vi "GetParticleResultValue.vi"(8 "error in (no error)":errorcluster, 9 "Data":T1, 11 "Analysis_Particle_Parameter":T2={"Selected Particle"=0, "Connectivity 4/8 (8)"=TRUE, "MaxParticle"=0}) -> (0 "error out":errorcluster, 3 "ResultValues":string[](array[string]))   [LabVIEW 2019]
uses:
  Controls/Particle/Analysis_Particle_Parameter.ctl
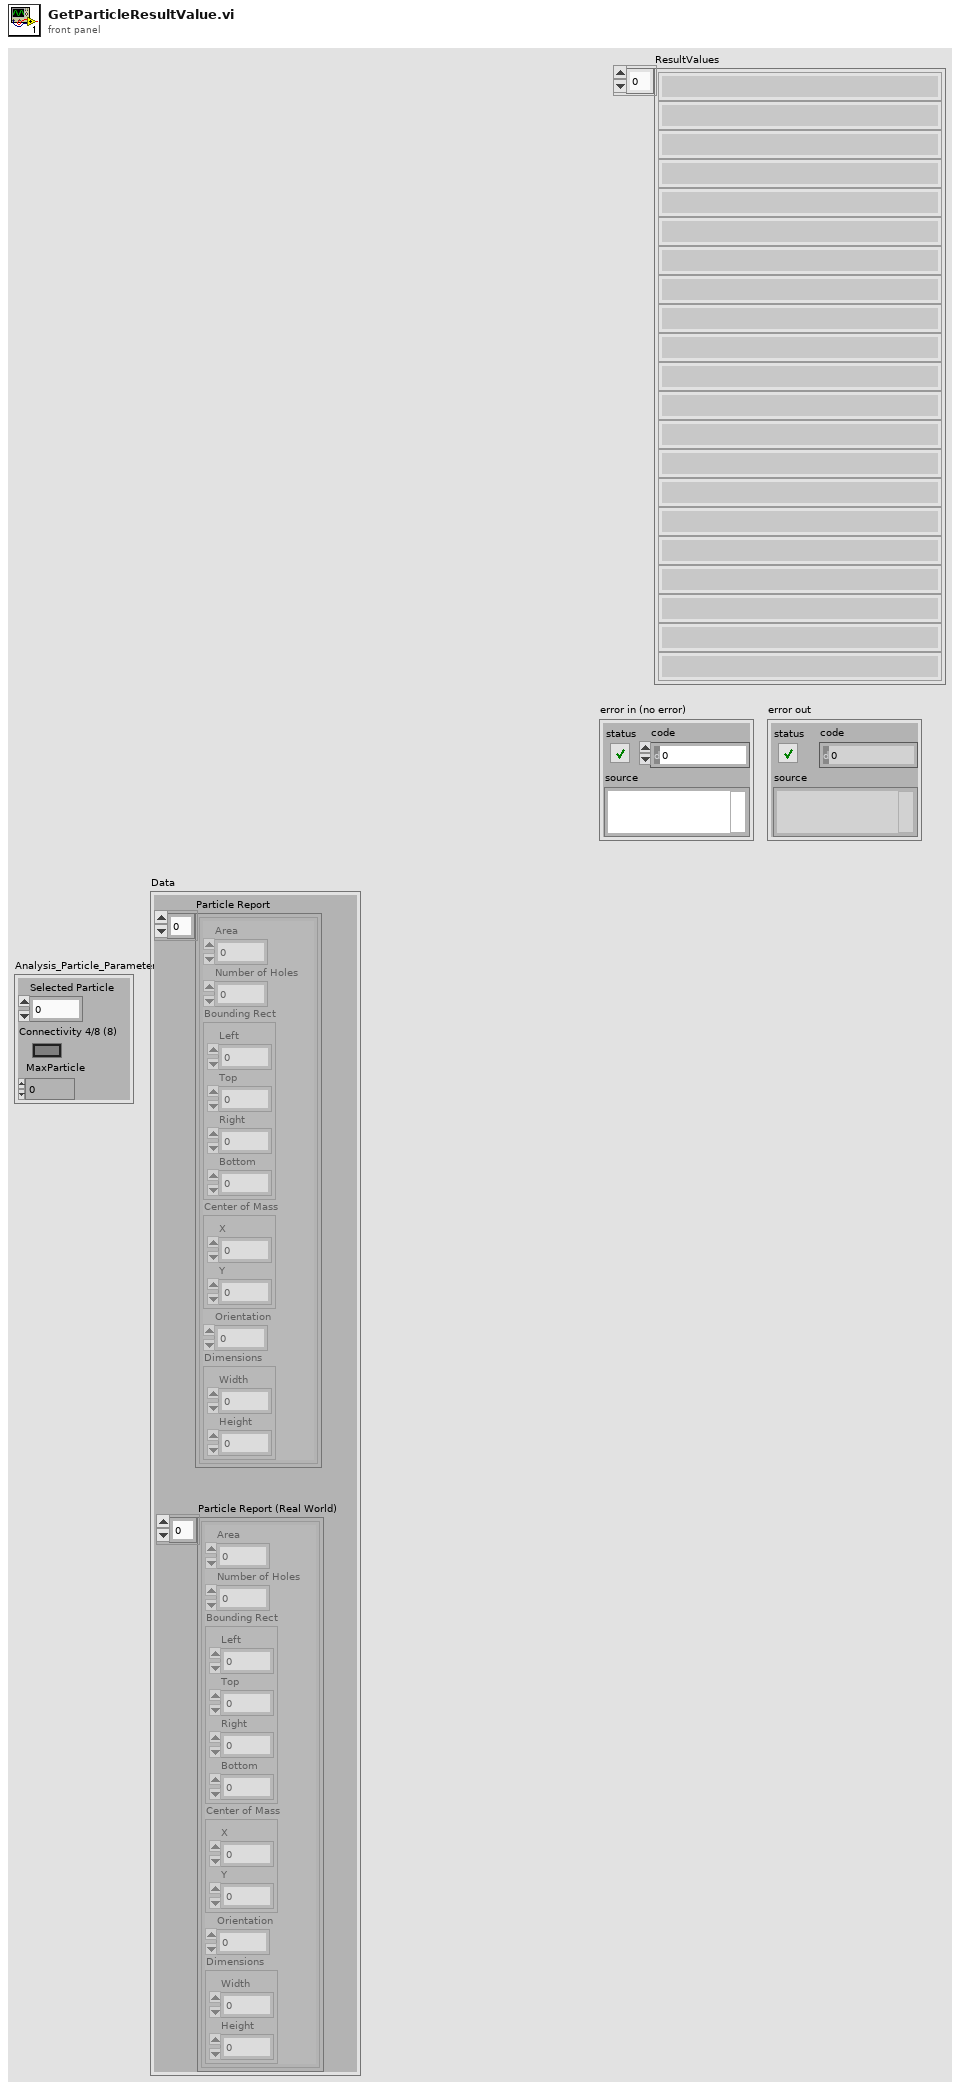
[diagram p1: front panel]
types:
  T1 = cluster{"Particle Report":cluster{"Area":dbl, "Number of Holes":dbl, "Bounding Rect":cluster{"Left":dbl, "Top":dbl, "Right":dbl, "Bottom":dbl}, "Center of Mass":cluster{"X":dbl, "Y":dbl}, "Orientation":dbl, "Dimensions":cluster{"Width":dbl, "Height":dbl}}[], "Particle Report (Real World)":cluster{"Area":dbl, "Number of Holes":dbl, "Bounding Rect":cluster{"Left":dbl, "Top":dbl, "Right":dbl, "Bottom":dbl}, "Center of Mass":cluster{"X":dbl, "Y":dbl}, "Orientation":dbl, "Dimensions":cluster{"Width":dbl, "Height":dbl}}[]}
  T2 = typedef "Analysis_Particle_Parameter.ctl" = cluster{"Selected Particle":i32, "Connectivity 4/8 (8)":bool, "MaxParticle":i32}
  T3 = cluster{"Area":dbl, "Number of Holes":dbl, "Bounding Rect":cluster{"Left":dbl, "Top":dbl, "Right":dbl, "Bottom":dbl}, "Center of Mass":cluster{"X":dbl, "Y":dbl}, "Orientation":dbl, "Dimensions":cluster{"Width":dbl, "Height":dbl}}[]
  T4 = cluster{"Left":dbl, "Top":dbl, "Right":dbl, "Bottom":dbl}
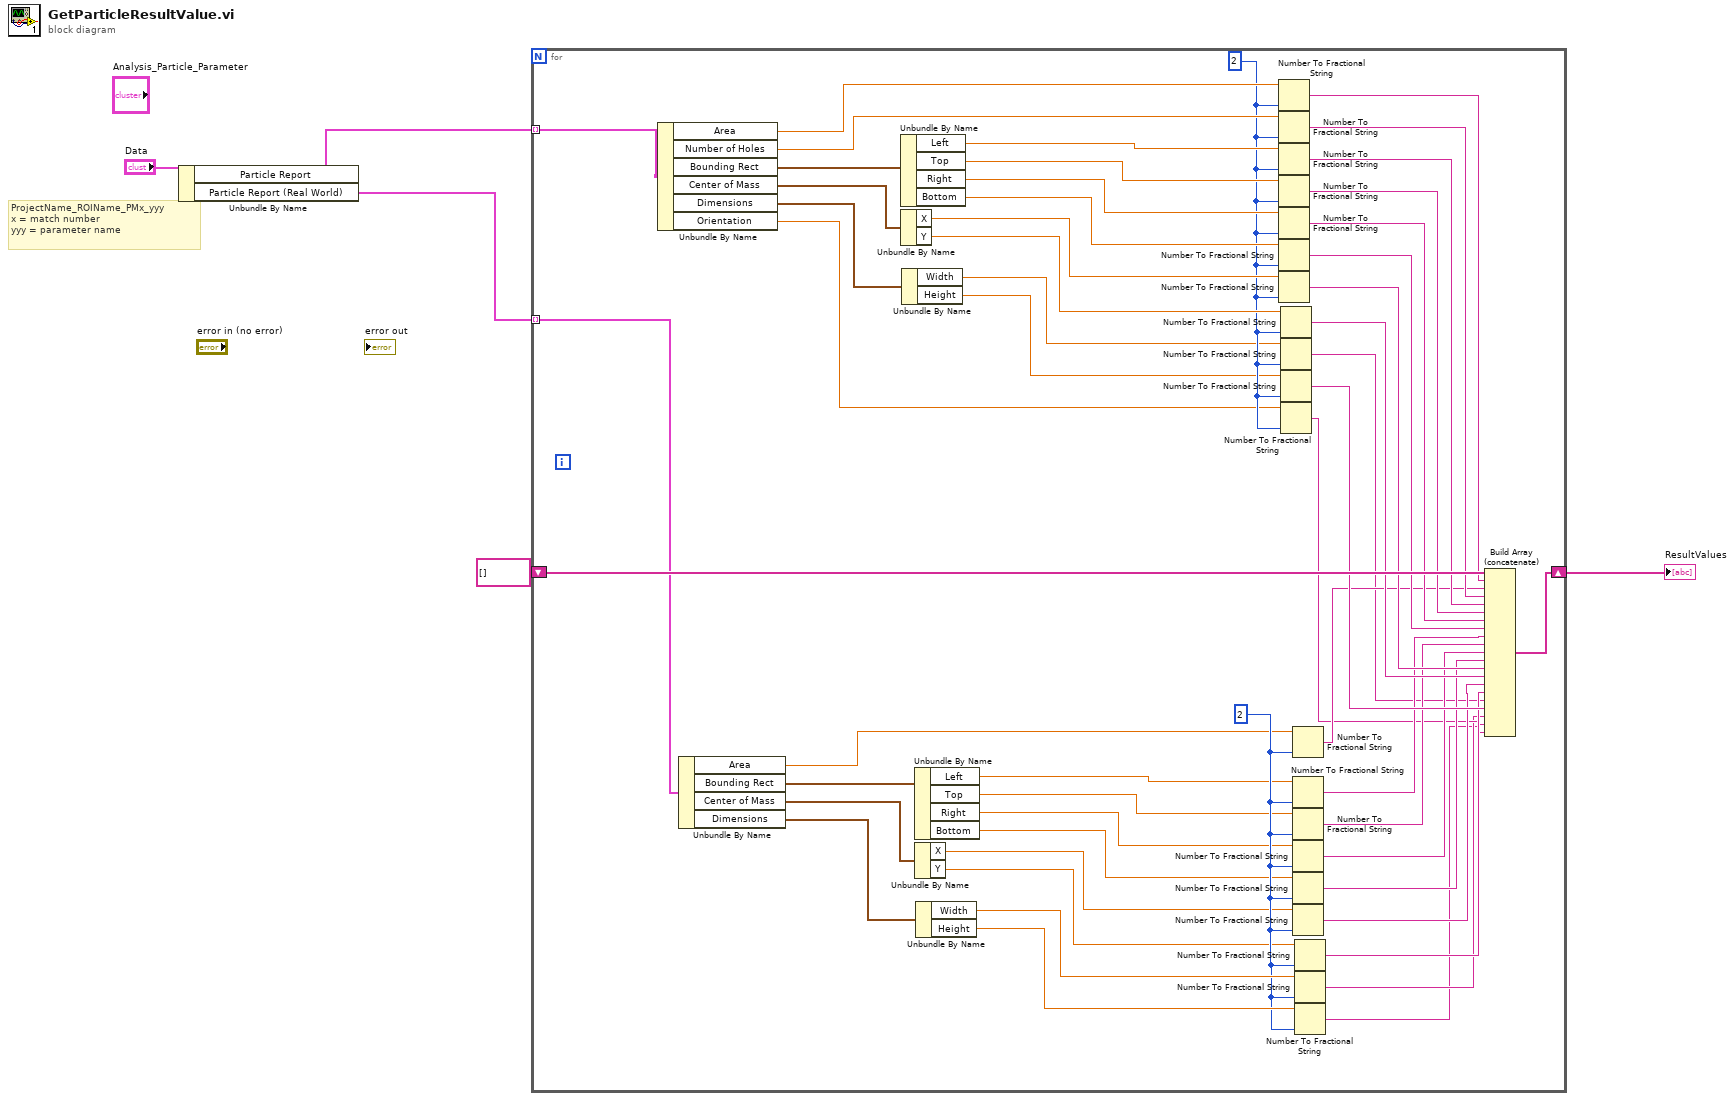
[diagram p0: block diagram]
diagram:
  # "ProjectName_ROIName_PMx_yyy\nx = match number\nyyy = parameter name"
  n1 = Unbundle By Name("Data") -> ("Particle Report"=w2:T3, "Particle Report (Real World)"=w1:T3)
  n2 = for {
    shift-right: [w31] -> w4
    shift-left: string[] [] -> [w57]
    tunnel: w2 -> [w41] mode=indexing
    tunnel: w1 -> [w17] mode=indexing
    w27 = 2
    w46 = 2
    n3 = Unbundle By Name(w41) -> ("Area"=w54:dbl, "Number of Holes"=w53:dbl, "Bounding Rect"=w56:T4, "Center of Mass"=w55:cluster{"X":dbl, "Y":dbl}, "Dimensions"=w45:cluster{"Width":dbl, "Height":dbl}, "Orientation"=w42:dbl)
    n4 = Unbundle By Name(w17) -> ("Area"=w20:dbl, "Bounding Rect"=w18:T4, "Center of Mass"=w19:cluster{"X":dbl, "Y":dbl}, "Dimensions"=w28:cluster{"Width":dbl, "Height":dbl})
    n5 = Unbundle By Name(w56) -> ("Left"=w52:dbl, "Top"=w51:dbl, "Right"=w50:dbl, "Bottom"=w49:dbl)
    n6 = Unbundle By Name(w55) -> ("X"=w48:dbl, "Y"=w47:dbl)
    n7 = Unbundle By Name(w45) -> ("Width"=w44:dbl, "Height"=w43:dbl)
    n8 = Unbundle By Name(w18) -> ("Left"=w21:dbl, "Top"=w22:dbl, "Right"=w23:dbl, "Bottom"=w24:dbl)
    n9 = Unbundle By Name(w19) -> ("X"=w25:dbl, "Y"=w26:dbl)
    n10 = Unbundle By Name(w28) -> ("Width"=w29:dbl, "Height"=w30:dbl)
    n11 = Number To Fractional String(number=w54, precision (6)=w46) -> (F-format string=w40:string)  [unwired: 2 in]
    n12 = Number To Fractional String(number=w53, precision (6)=w46) -> (F-format string=w39:string)  [unwired: 2 in]
    n13 = Number To Fractional String(number=w52, precision (6)=w46) -> (F-format string=w38:string)  [unwired: 2 in]
    n14 = Number To Fractional String(number=w51, precision (6)=w46) -> (F-format string=w37:string)  [unwired: 2 in]
    n15 = Number To Fractional String(number=w50, precision (6)=w46) -> (F-format string=w36:string)  [unwired: 2 in]
    n16 = Number To Fractional String(number=w49, precision (6)=w46) -> (F-format string=w35:string)  [unwired: 2 in]
    n17 = Number To Fractional String(number=w48, precision (6)=w46) -> (F-format string=w34:string)  [unwired: 2 in]
    n18 = Number To Fractional String(number=w47, precision (6)=w46) -> (F-format string=w33:string)  [unwired: 2 in]
    n19 = Number To Fractional String(number=w44, precision (6)=w46) -> (F-format string=w9:string)  [unwired: 2 in]
    n20 = Number To Fractional String(number=w43, precision (6)=w46) -> (F-format string=w32:string)  [unwired: 2 in]
    n21 = Number To Fractional String(number=w42, precision (6)=w46) -> (F-format string=w8:string)  [unwired: 2 in]
    n22 = Number To Fractional String(number=w20, precision (6)=w27) -> (F-format string=w16:string)  [unwired: 2 in]
    n23 = Number To Fractional String(number=w21, precision (6)=w27) -> (F-format string=w15:string)  [unwired: 2 in]
    n24 = Number To Fractional String(number=w22, precision (6)=w27) -> (F-format string=w14:string)  [unwired: 2 in]
    n25 = Number To Fractional String(number=w23, precision (6)=w27) -> (F-format string=w13:string)  [unwired: 2 in]
    n26 = Number To Fractional String(number=w24, precision (6)=w27) -> (F-format string=w12:string)  [unwired: 2 in]
    n27 = Number To Fractional String(number=w25, precision (6)=w27) -> (F-format string=w11:string)  [unwired: 2 in]
    n28 = Number To Fractional String(number=w26, precision (6)=w27) -> (F-format string=w10:string)  [unwired: 2 in]
    n29 = Number To Fractional String(number=w29, precision (6)=w27) -> (F-format string=w7:string)  [unwired: 2 in]
    n30 = Number To Fractional String(number=w30, precision (6)=w27) -> (F-format string=w6:string)  [unwired: 2 in]
    n31 = Build Array (concatenate)(w57, w40, w16, w39, w38, w37, w36, w35, w15, w14, w13, w12, w34, w33, w11, w10, w9, w32, w7, w6, w8) -> (w31:string[])
  }
  "ResultValues" <- w4
